vi "test-swerve-drve-odometry-03.vi"() -> (3 "Test Passed":bool)   [LabVIEW 2019]
uses:
  <vilib>/Rock Robotics/WPI/ThirdParty/JAS_Junk/TrajLib/SWERVE_DRIVE_ODOMETRY.ctl
  <vilib>/Rock Robotics/WPI/ThirdParty/JAS_Junk/TrajLib/POSE2D.ctl
  <vilib>/Rock Robotics/WPI/ThirdParty/JAS_Junk/TrajLib/TRANSLATION2D.ctl
  <vilib>/Rock Robotics/WPI/ThirdParty/JAS_Junk/TrajLib/ROTATION2D.ctl
  <vilib>/Rock Robotics/WPI/ThirdParty/JAS_Junk/TrajLib/SWERVE_DRIVE_KINEMATICS.ctl
  <vilib>/Analysis/Matrix/Datatypes/RealMatrix.ctl
  <vilib>/Rock Robotics/WPI/ThirdParty/JAS_Junk/TrajLib/Conv_Deg_Radians.vi
  <vilib>/Rock Robotics/WPI/ThirdParty/JAS_Junk/TrajLib/Rotation2d_CreateAngle.vi
  <vilib>/Rock Robotics/WPI/ThirdParty/JAS_Junk/TrajLib/Trajectory_Library.lvlib
  <vilib>/Analysis/Matrix/NI_Matrix.lvlib
panel:
  out "SWERVE_DRIVE_KINEMATICS":T1 {"PrevCoR"."Y" format="%14.3f"; "PrevCoR"."X" format="%14.3f"; "Modules"."Y" format="%14.3f"; "Modules"."X" format="%14.3f"}
  out "robot POSE 3":T4={"TRANSLATION"={"X"=0.0, "Y"=0.0}, "ROTATION"={"VALUE"=0.0, "COS"=1.0, "SIN"=0.0}} {"ROTATION"."SIN" format="%13.4f"; "ROTATION"."COS" format="%13.4f"; "ROTATION"."VALUE" format="%13.4f"; "TRANSLATION"."Y" format="%14.3f"; "TRANSLATION"."X" format="%14.3f"}
  out "Odom 3":T6={"POSE"={"TRANSLATION"={"X"=0.0, "Y"=0.0}, "ROTATION"={"VALUE"=0.0, "COS"=1.0, "SIN"=0.0}}, "GyroOffset"={"VALUE"=0.0, "COS"=1.0, "SIN"=0.0}, "PreviousAngle"={"VALUE"=0.0, "COS"=1.0, "SIN"=0.0}, "PrevTime"=0.0} {"PreviousAngle"."SIN" format="%13.4f"; "PreviousAngle"."COS" format="%13.4f"; "PreviousAngle"."VALUE" format="%13.4f"; "GyroOffset"."SIN" format="%13.4f"; "GyroOffset"."COS" format="%13.4f"; "GyroOffset"."VALUE" format="%13.4f"; "POSE"."ROTATION"."SIN" format="%13.4f"; "POSE"."ROTATION"."COS" format="%13.4f"; "POSE"."ROTATION"."VALUE" format="%13.4f"; "POSE"."TRANSLATION"."Y" format="%14.3f"; "POSE"."TRANSLATION"."X" format="%14.3f"}
  out "Odom 1":T6={"POSE"={"TRANSLATION"={"X"=0.0, "Y"=0.0}, "ROTATION"={"VALUE"=0.0, "COS"=1.0, "SIN"=0.0}}, "GyroOffset"={"VALUE"=0.0, "COS"=1.0, "SIN"=0.0}, "PreviousAngle"={"VALUE"=0.0, "COS"=1.0, "SIN"=0.0}, "PrevTime"=0.0} {"PreviousAngle"."SIN" format="%13.4f"; "PreviousAngle"."COS" format="%13.4f"; "PreviousAngle"."VALUE" format="%13.4f"; "GyroOffset"."SIN" format="%13.4f"; "GyroOffset"."COS" format="%13.4f"; "GyroOffset"."VALUE" format="%13.4f"; "POSE"."ROTATION"."SIN" format="%13.4f"; "POSE"."ROTATION"."COS" format="%13.4f"; "POSE"."ROTATION"."VALUE" format="%13.4f"; "POSE"."TRANSLATION"."Y" format="%14.3f"; "POSE"."TRANSLATION"."X" format="%14.3f"}
  out "Odom 0":T6={"POSE"={"TRANSLATION"={"X"=0.0, "Y"=0.0}, "ROTATION"={"VALUE"=0.0, "COS"=1.0, "SIN"=0.0}}, "GyroOffset"={"VALUE"=0.0, "COS"=1.0, "SIN"=0.0}, "PreviousAngle"={"VALUE"=0.0, "COS"=1.0, "SIN"=0.0}, "PrevTime"=0.0} {"PreviousAngle"."SIN" format="%13.4f"; "PreviousAngle"."COS" format="%13.4f"; "PreviousAngle"."VALUE" format="%13.4f"; "GyroOffset"."SIN" format="%13.4f"; "GyroOffset"."COS" format="%13.4f"; "GyroOffset"."VALUE" format="%13.4f"; "POSE"."ROTATION"."SIN" format="%13.4f"; "POSE"."ROTATION"."COS" format="%13.4f"; "POSE"."ROTATION"."VALUE" format="%13.4f"; "POSE"."TRANSLATION"."Y" format="%14.3f"; "POSE"."TRANSLATION"."X" format="%14.3f"}
  out "robot POSE 0":T4={"TRANSLATION"={"X"=0.0, "Y"=0.0}, "ROTATION"={"VALUE"=0.0, "COS"=1.0, "SIN"=0.0}} {"ROTATION"."SIN" format="%13.4f"; "ROTATION"."COS" format="%13.4f"; "ROTATION"."VALUE" format="%13.4f"; "TRANSLATION"."Y" format="%14.3f"; "TRANSLATION"."X" format="%14.3f"}
  out "robot POSE 2":T4={"TRANSLATION"={"X"=0.0, "Y"=0.0}, "ROTATION"={"VALUE"=0.0, "COS"=1.0, "SIN"=0.0}} {"ROTATION"."SIN" format="%13.4f"; "ROTATION"."COS" format="%13.4f"; "ROTATION"."VALUE" format="%13.4f"; "TRANSLATION"."Y" format="%14.3f"; "TRANSLATION"."X" format="%14.3f"}
  out "Odom 2":T6={"POSE"={"TRANSLATION"={"X"=0.0, "Y"=0.0}, "ROTATION"={"VALUE"=0.0, "COS"=1.0, "SIN"=0.0}}, "GyroOffset"={"VALUE"=0.0, "COS"=1.0, "SIN"=0.0}, "PreviousAngle"={"VALUE"=0.0, "COS"=1.0, "SIN"=0.0}, "PrevTime"=0.0} {"PreviousAngle"."SIN" format="%13.4f"; "PreviousAngle"."COS" format="%13.4f"; "PreviousAngle"."VALUE" format="%13.4f"; "GyroOffset"."SIN" format="%13.4f"; "GyroOffset"."COS" format="%13.4f"; "GyroOffset"."VALUE" format="%13.4f"; "POSE"."ROTATION"."SIN" format="%13.4f"; "POSE"."ROTATION"."COS" format="%13.4f"; "POSE"."ROTATION"."VALUE" format="%13.4f"; "POSE"."TRANSLATION"."Y" format="%14.3f"; "POSE"."TRANSLATION"."X" format="%14.3f"}
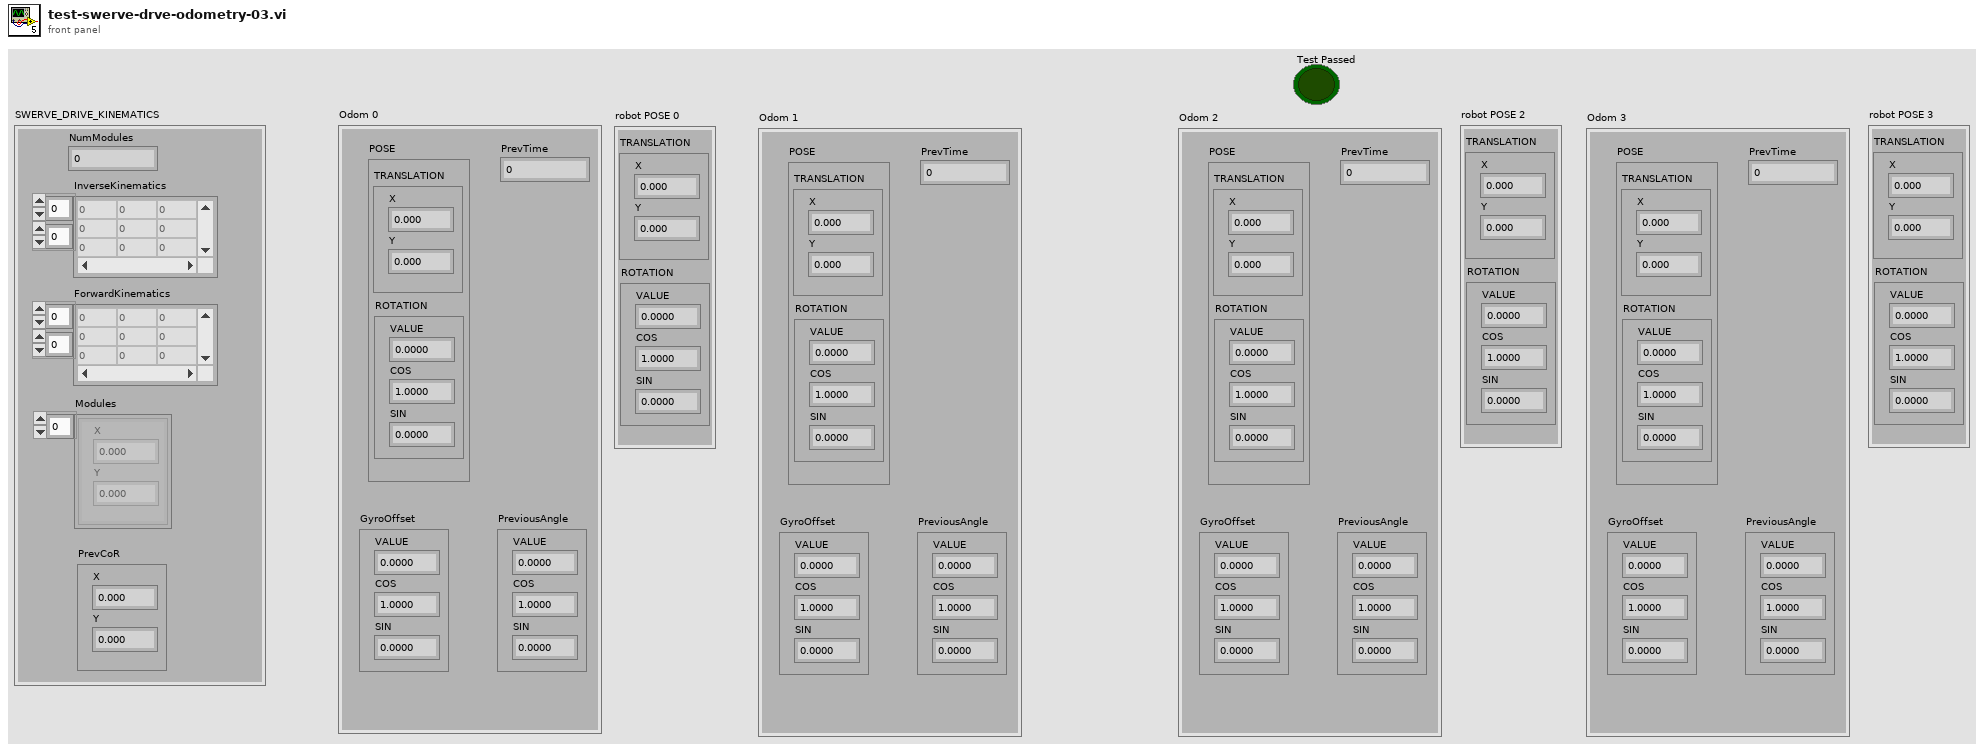
[diagram p1: front panel]
types:
  T1 = typedef "Trajectory_Library.lvlib/SWERVE_DRIVE_KINEMATICS.ctl" = cluster{"NumModules":i32, "InverseKinematics":T2, "ForwardKinematics":T2, "Modules":T3[], "PrevCoR":T3}
  T2 = typedef "NI_Matrix.lvlib/RealMatrix.ctl" = dbl[][]
  T3 = typedef "Trajectory_Library.lvlib/TRANSLATION2D.ctl" = cluster{"X":dbl, "Y":dbl}
  T4 = typedef "Trajectory_Library.lvlib/POSE2D.ctl" = cluster{"TRANSLATION":T3, "ROTATION":T5}
  T5 = typedef "Trajectory_Library.lvlib/ROTATION2D.ctl" = cluster{"VALUE":dbl, "COS":dbl, "SIN":dbl}
  T6 = typedef "Trajectory_Library.lvlib/SWERVE_DRIVE_ODOMETRY.ctl" = cluster{"POSE":T4, "GyroOffset":T5, "PreviousAngle":T5, "PrevTime":dbl}
  T7 = typedef "Trajectory_Library.lvlib/SWERVE_DRIVE_MODULE_STATE.ctl" = cluster{"Speed":dbl, "Angle":T5}
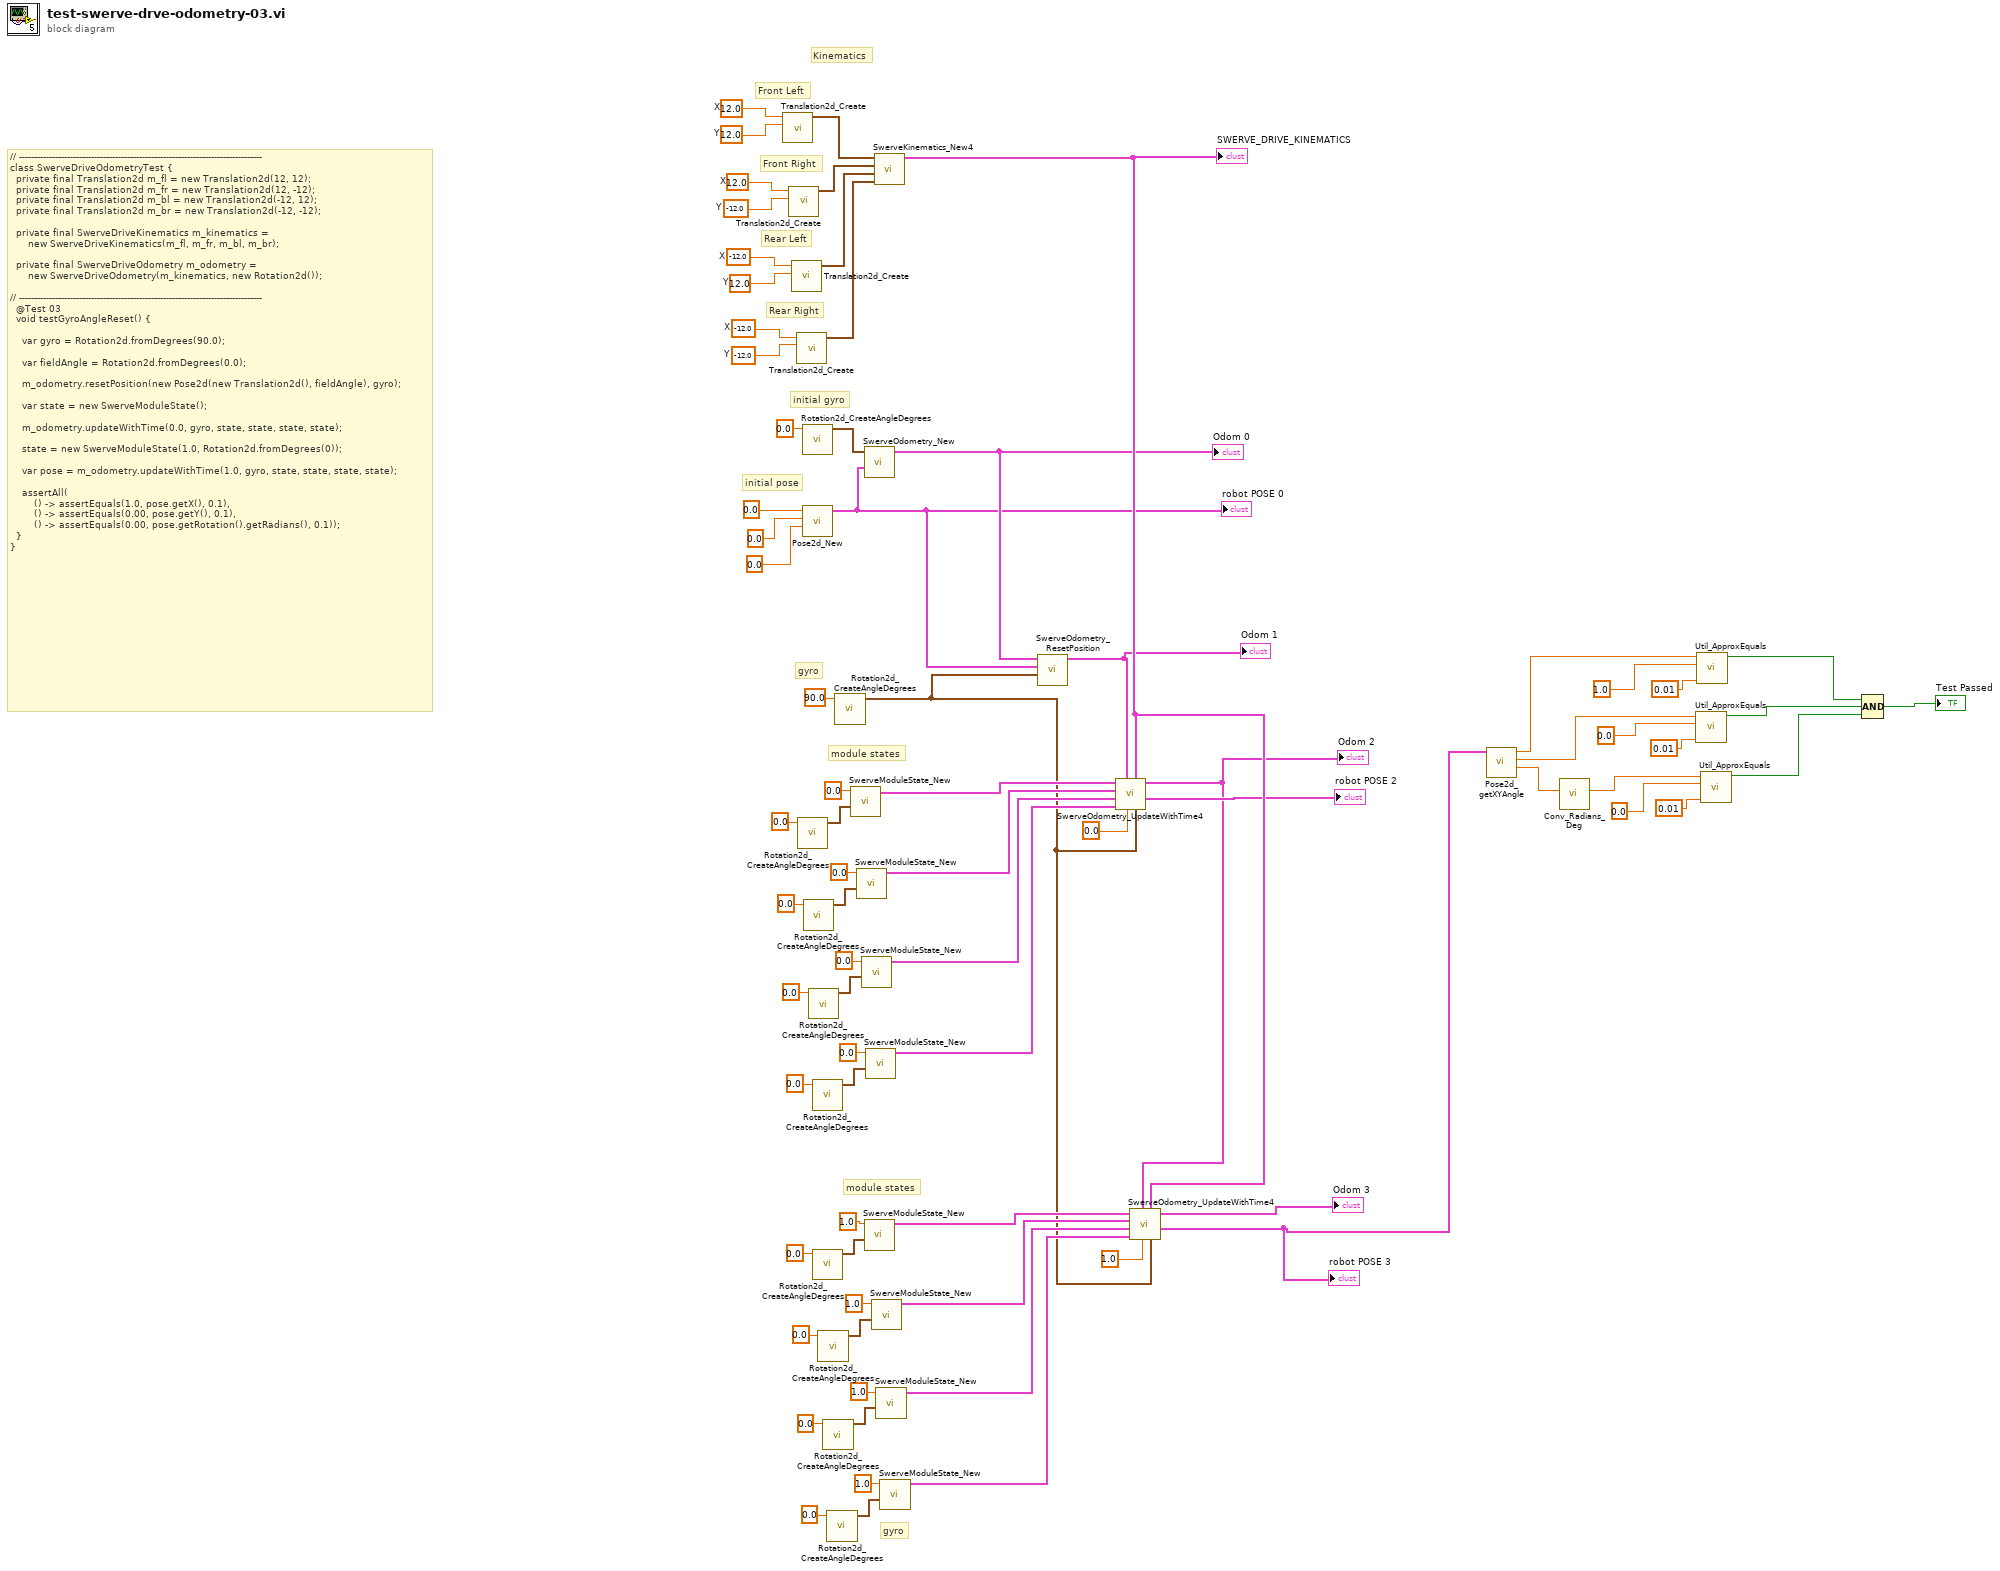
[diagram p0: block diagram]
diagram:
  w71 = -12.0  # X
  w70 = -12.0  # Y
  w69 = -12.0  # X
  w68 = 12.0  # Y
  w67 = 12.0  # X
  w66 = -12.0  # Y
  w65 = 12.0  # X
  w64 = 12.0  # Y
  # "gyro"
  # "initial pose"
  # "gyro"
  # "module states"
  # "module states"
  # "Kinematics"
  # "initial gyro"
  # "Rear Right"
  # "Rear Left"
  # "Front Right"
  # "Front Left"
  # "// ---------------------------------------------------------------------------------\nclass SwerveDriveOdometryTest {\n  private final Translation2d m_fl = new Translation2d(12, 12);\n  private final Translation2d m_fr = new Translation2d(12, -12);\n  private final Translation2d m_bl = new Translation2d(-12, 12);\n  private final Translation2d m_br = new Translation2d(-12, -12);\n\n  private final SwerveDriveKinematics m_kinematics =\n      new SwerveDriveKinematics(m_fl, m_fr, m_bl, m_br);\n\n  private final SwerveDriveOdometry m_odometry =\n      new SwerveDriveOdometry(m_kinematics, new Rotation2d());\n\n// ---------------------------------------------------------------------------------\n  @Test 03\n  void testGyroAngleReset() {\n\n    var gyro = Rotation2d.fromDegrees(90.0);\n\n    var fieldAngle = Rotation2d.fromDegrees(0.0);\n\n    m_odometry.resetPosition(new Pose2d(new Translation2d(), fieldAngle), gyro);\n\n    var state = new SwerveModuleState();\n\n    m_odometry.updateWithTime(0.0, gyro, state, state, state, state);\n\n    state = new SwerveModuleState(1.0, Rotation2d.fromDegrees(0));\n\n    var pose = m_odometry.updateWithTime(1.0, gyro, state, state, state, state);\n\n    assertAll(\n        () -> assertEquals(1.0, pose.getX(), 0.1),\n        () -> assertEquals(0.00, pose.getY(), 0.1),\n        () -> assertEquals(0.00, pose.getRotation().getRadians(), 0.1));\n  }\n}"
  n1 = call <vilib>:"Translation2d_Create.vi"("Y"=w64, "X"=w65) -> ("TRANSLATION"=w72:T3)  [unwired: 9 in]
  n2 = call <vilib>:"Translation2d_Create.vi"("Y"=w66, "X"=w67) -> ("TRANSLATION"=w73:T3)  [unwired: 9 in]
  n3 = call <vilib>:"Translation2d_Create.vi"("Y"=w68, "X"=w69) -> ("TRANSLATION"=w74:T3)  [unwired: 9 in]
  n4 = call <vilib>:"Translation2d_Create.vi"("Y"=w70, "X"=w71) -> ("TRANSLATION"=w75:T3)  [unwired: 9 in]
  n5 = call <vilib>:"Rotation2d_CreateAngleDegrees.vi"("Angle_Degrees"=0.0) -> ("ROTATION"=w57:T5)  [unwired: 10 in]
  n6 = call <vilib>:"Rotation2d_CreateAngleDegrees.vi"("Angle_Degrees"=0.0) -> ("ROTATION"=w60:T5)  [unwired: 10 in]
  n7 = call <vilib>:"Pose2d_New.vi"("Heading"=0.0, "Y"=0.0, "X"=0.0) -> ("out POSe"=w4:T4)  [unwired: 8 in]
  "robot POSE 0" <- w4
  n8 = call <vilib>:"Rotation2d_CreateAngleDegrees.vi"("Angle_Degrees"=0.0) -> ("ROTATION"=w54:T5)  [unwired: 10 in]
  n9 = call <vilib>:"Rotation2d_CreateAngleDegrees.vi"("Angle_Degrees"=0.0) -> ("ROTATION"=w51:T5)  [unwired: 10 in]
  n10 = call <vilib>:"Rotation2d_CreateAngleDegrees.vi"("Angle_Degrees"=0.0) -> ("ROTATION"=w48:T5)  [unwired: 10 in]
  n11 = call <vilib>:"Rotation2d_CreateAngleDegrees.vi"("Angle_Degrees"=0.0) -> ("ROTATION"=w41:T5)  [unwired: 10 in]
  n12 = call <vilib>:"Rotation2d_CreateAngleDegrees.vi"("Angle_Degrees"=0.0) -> ("ROTATION"=w38:T5)  [unwired: 10 in]
  n13 = call <vilib>:"Rotation2d_CreateAngleDegrees.vi"("Angle_Degrees"=0.0) -> ("ROTATION"=w35:T5)  [unwired: 10 in]
  n14 = call <vilib>:"Rotation2d_CreateAngleDegrees.vi"("Angle_Degrees"=0.0) -> ("ROTATION"=w32:T5)  [unwired: 10 in]
  n15 = call <vilib>:"Rotation2d_CreateAngleDegrees.vi"("Angle_Degrees"=90.0) -> ("ROTATION"=w3:T5)  [unwired: 10 in]
  n16 = call <vilib>:"SwerveModuleState_New.vi"("ROTATION"=w57, "Speed"=0.0) -> ("SWERVE_DRIVE_MODULE_STATE"=w46:T7)  [unwired: 9 in]
  n17 = call <vilib>:"SwerveModuleState_New.vi"("ROTATION"=w54, "Speed"=0.0) -> ("SWERVE_DRIVE_MODULE_STATE"=w45:T7)  [unwired: 9 in]
  n18 = call <vilib>:"SwerveModuleState_New.vi"("ROTATION"=w51, "Speed"=0.0) -> ("SWERVE_DRIVE_MODULE_STATE"=w44:T7)  [unwired: 9 in]
  n19 = call <vilib>:"SwerveOdometry_New.vi"("InitialPose"=w4, "gyroAngle"=w60) -> ("SWERVE_DRIVE_ODOMETRY"=w9:T6)  [unwired: 9 in]
  "Odom 0" <- w9
  n20 = call <vilib>:"SwerveModuleState_New.vi"("ROTATION"=w41, "Speed"=1.0) -> ("SWERVE_DRIVE_MODULE_STATE"=w30:T7)  [unwired: 9 in]
  n21 = call <vilib>:"SwerveModuleState_New.vi"("ROTATION"=w48, "Speed"=0.0) -> ("SWERVE_DRIVE_MODULE_STATE"=w43:T7)  [unwired: 9 in]
  n22 = call <vilib>:"SwerveModuleState_New.vi"("ROTATION"=w38, "Speed"=1.0) -> ("SWERVE_DRIVE_MODULE_STATE"=w29:T7)  [unwired: 9 in]
  n23 = call <vilib>:"SwerveKinematics_New4.vi"("wheel 3"=w75, "wheel 2"=w74, "wheel 1"=w73, "wheel 0"=w72) -> ("SWERVE_DRIVE_KINEMATICS"=w24:T1)  [unwired: 7 in]
  "SWERVE_DRIVE_KINEMATICS" <- w24
  n24 = call <vilib>:"SwerveModuleState_New.vi"("ROTATION"=w35, "Speed"=1.0) -> ("SWERVE_DRIVE_MODULE_STATE"=w28:T7)  [unwired: 9 in]
  n25 = call <vilib>:"SwerveModuleState_New.vi"("ROTATION"=w32, "Speed"=1.0) -> ("SWERVE_DRIVE_MODULE_STATE"=w27:T7)  [unwired: 9 in]
  n26 = call <vilib>:"SwerveOdometry_ResetPosition.vi"("gyroAngle"=w3, "Pose"=w4, "in SWERVE_DRIVE_ODOMETRY"=w9) -> ("out SWERVE_DRIVE_ODOMETRY"=w8:T6)  [unwired: 8 in]
  "Odom 1" <- w8
  n27 = call <vilib>:"SwerveOdometry_UpdateWithTime4.vi"("gyroAngle"=w3, "SWERVE_DRIVE_KINEMATICS"=w24, "Time"=0.0, "in SWERVE_DRIVE_ODOMETRY"=w8, "Wheel State 3"=w43, "Wheel State 2"=w44, "Wheel State 1"=w45, "Wheel State 0"=w46) -> ("robot POSE"=→"robot POSE 2":T4, "out SWERVE_DRIVE_ODOMETRY"=w6:T6)  [unwired: 2 in]
  "Odom 2" <- w6
  n28 = call <vilib>:"SwerveOdometry_UpdateWithTime4.vi"("gyroAngle"=w3, "SWERVE_DRIVE_KINEMATICS"=w24, "Time"=1.0, "in SWERVE_DRIVE_ODOMETRY"=w6, "Wheel State 3"=w27, "Wheel State 2"=w28, "Wheel State 1"=w29, "Wheel State 0"=w30) -> ("robot POSE"=w1:T4, "out SWERVE_DRIVE_ODOMETRY"=→"Odom 3":T6)  [unwired: 2 in]
  "robot POSE 3" <- w1
  n29 = call <vilib>:"Pose2d_getXYAngle.vi"("in POSE"=w1) -> ("Angle"=w20:dbl, "Y"=w18:dbl, "X"=w19:dbl)  [unwired: 8 in]
  n30 = call <vilib>:"Conv_Radians_Deg.vi"("Radians"=w20) -> ("Degrees"=w17:dbl)  [unwired: 10 in]
  n31 = call <vilib>:"Util_ApproxEquals.vi"("Tolerance"=0.01, "Value 2"=0.0, "Value 1"=w18) -> ("ApproxEquals"=w12:bool)  [unwired: 8 in]
  n32 = call <vilib>:"Util_ApproxEquals.vi"("Tolerance"=0.01, "Value 2"=1.0, "Value 1"=w19) -> ("ApproxEquals"=w13:bool)  [unwired: 8 in]
  n33 = call <vilib>:"Util_ApproxEquals.vi"("Tolerance"=0.01, "Value 2"=0.0, "Value 1"=w17) -> ("ApproxEquals"=w11:bool)  [unwired: 8 in]
  n34 = Compound Arithmetic op=AND(w13, w12, w11) -> (→"Test Passed":bool)
